vi "Vacuum Configuration to Strings.vi"(11 "Test Information":T1) -> (2 "Thresholds":string[][](array[string]), 3 "Timings":string[][](array[string]))   [LabVIEW 2015]
uses:
  Tests/Controls/Test Information.ctl
  Tests/Controls/Vacuum Test.ctl
  Tests/Controls/Test Timing.ctl
  Tests/Controls/Vaccum Thresholds.ctl
  Tests/Controls/Helium Test.ctl
  Tests/Controls/Helium Thresholds.ctl
  Tests/Controls/Startup Thresholds.ctl
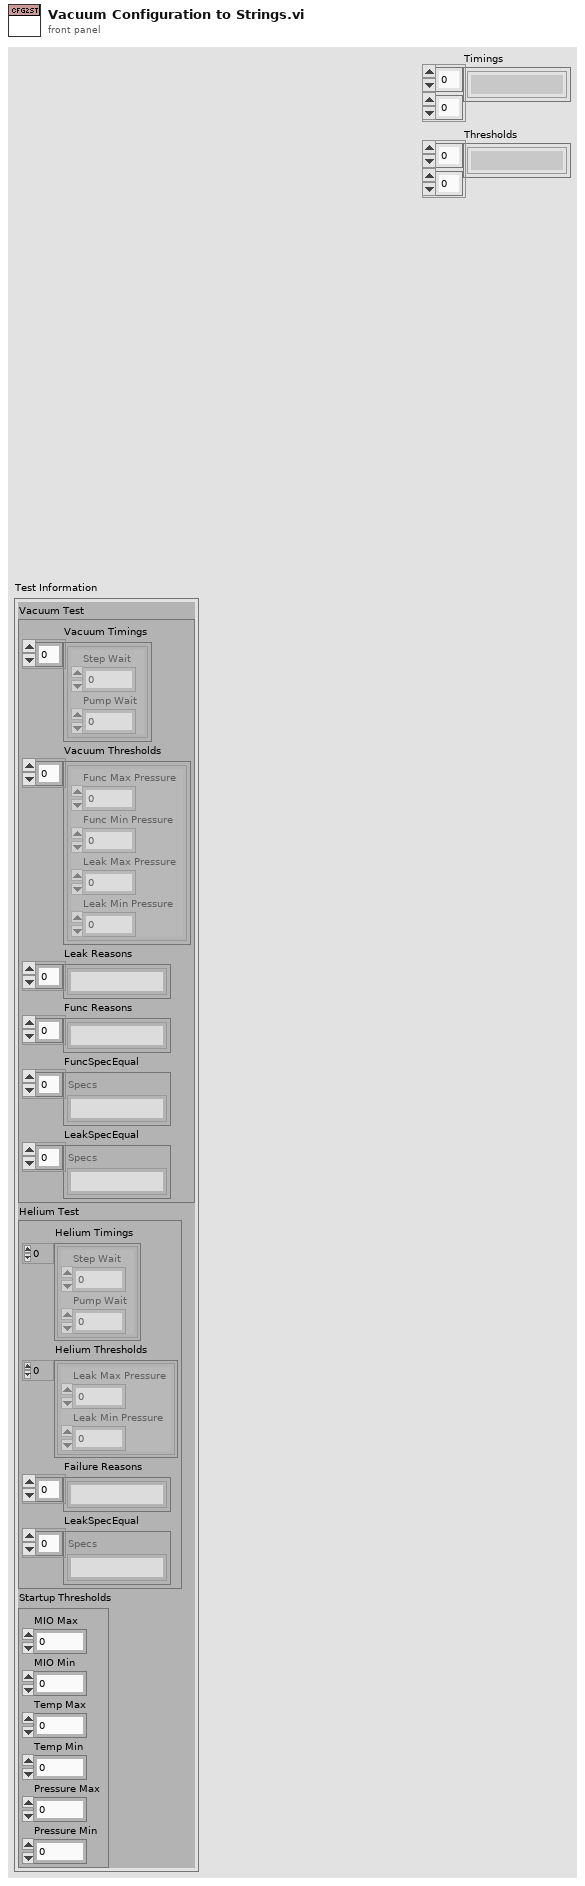
[diagram p1: front panel]
types:
  T1 = typedef "Test Information.ctl" = cluster{"Vacuum Test":T2, "Helium Test":T5, "Startup Thresholds":T7}
  T2 = typedef "Vacuum Test.ctl" = cluster{"Vacuum Timings":T3[], "Vacuum Thresholds":T4[], "Leak Reasons":string[], "Func Reasons":string[], "FuncSpecEqual":string[], "LeakSpecEqual":string[]}
  T3 = typedef "Test Timing.ctl" = cluster{"Step Wait":dbl, "Pump Wait":dbl}
  T4 = typedef "Vaccum Thresholds.ctl" = cluster{"Func Max Pressure":dbl, "Func Min Pressure":dbl, "Leak Max Pressure":dbl, "Leak Min Pressure":dbl}
  T5 = typedef "Helium Test.ctl" = cluster{"Helium Timings":T3[], "Helium Thresholds":T6[], "Failure Reasons":string[], "LeakSpecEqual":string[]}
  T6 = typedef "Helium Thresholds.ctl" = cluster{"Leak Max Pressure":dbl, "Leak Min Pressure":dbl}
  T7 = typedef "Startup Thresholds.ctl" = cluster{"MIO Max":dbl, "MIO Min":dbl, "Temp Max":dbl, "Temp Min":dbl, "Pressure Max":dbl, "Pressure Min":dbl}
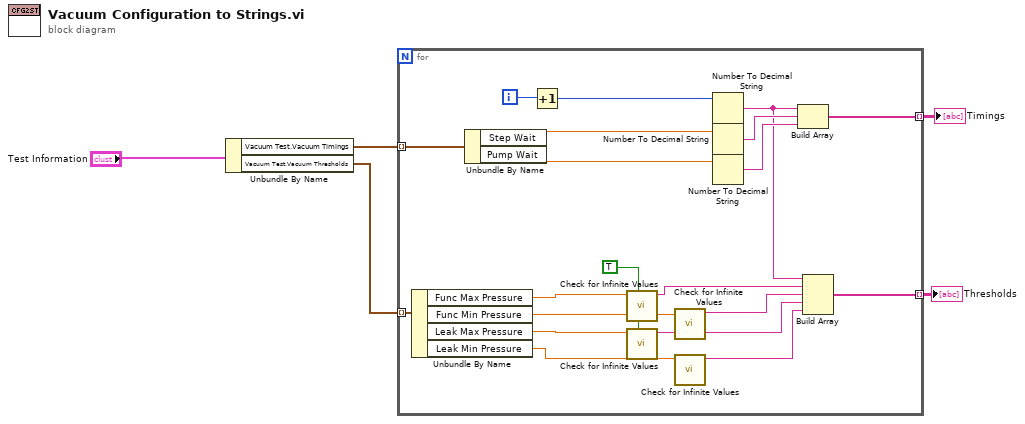
[diagram p0: block diagram]
diagram:
  n1 = Unbundle By Name("Test Information") -> ("Vacuum Test.Vacuum Timings"=w5:T3[], "Vacuum Test.Vacuum Thresholds"=w3:T4[])
  n2 = for {
    tunnel: w5 -> [w25] mode=indexing
    tunnel: [w22] -> w4 mode=indexing
    tunnel: w3 -> [w17] mode=indexing
    tunnel: [w15] -> w2 mode=indexing
    i -> [w24]
    w10 = TRUE ("Positive?")
    n3 = Unbundle By Name(w17) -> ("Func Max Pressure"=w14:dbl, "Func Min Pressure"=w12:dbl, "Leak Max Pressure"=w8:dbl, "Leak Min Pressure"=w9:dbl)
    n4 = Unbundle By Name(w25) -> ("Step Wait"=w21:dbl, "Pump Wait"=w20:dbl)
    n5 = Increment(x=w24) -> (x+1=w23:i32)
    n6 = call "Check for Infinite Values.vi"("Positive?"=w10, "Pressure Limit"=w14) -> ("element"=w13:string)  [unwired: 9 in]
    n7 = call "Check for Infinite Values.vi"("Positive?"=w10, "Pressure Limit"=w8) -> ("element"=w7:string)  [unwired: 9 in]
    n8 = call "Check for Infinite Values.vi"("Pressure Limit"=w12) -> ("element"=w11:string)  [unwired: 10 in]
    n9 = call "Check for Infinite Values.vi"("Pressure Limit"=w9) -> ("element"=w6:string)  [unwired: 10 in]
    n10 = Number To Decimal String(number=w23) -> (decimal integer string=w16:string)  [unwired: 1 in]
    n11 = Number To Decimal String(number=w21) -> (decimal integer string=w19:string)  [unwired: 1 in]
    n12 = Number To Decimal String(number=w20) -> (decimal integer string=w18:string)  [unwired: 1 in]
    n13 = Build Array(w16, w19, w18) -> (w22:string[])
    n14 = Build Array(w16, w13, w11, w7, w6) -> (w15:string[])
  }
  "Timings" <- w4
  "Thresholds" <- w2
